vi "Remote Access.vi"() -> ()   [LabVIEW 2020, in "Startup Processes.lvlib"]
uses:
  Startup Processes.lvlib
  toolbox/Standard Signalling/ude_Stop Application/ude_Stop Application.lvlib
  toolbox/Standard Signalling/ude_Handle Errors/ude_Handle Errors.lvlib
  _ude/Read Graph Data/Read Graph Data.lvlib
  toolbox/Standard Signalling/not_Generic Named Notifier/not_Generic Named Notifier.lvlib
  _buffers/Sine Signal Data Buffer/Sine Signal Data Buffer.lvlib
  _buffers/Ramp Signal Data Buffer/Ramp Signal Data Buffer.lvlib
  _buffers/Temperature Controller Data Buffer/Temperature Controller Data Buffer.lvlib
  _ude/Read Graph Image/Read Graph Image.lvlib
  _buffers/Plugin Chart References/Plugin Chart References.lvlib
  _ude/Set Acquisition Rate/Set Acquisition Rate.lvlib
  _buffers/Sample Rate/Sample Rate.lvlib
  _ude/Set Data Buffer Depth/Set Data Buffer Depth.lvlib
  _ude/Set TC Parameters/Set TC Parameters.lvlib
  Config Data/Config Data.lvclass
  _typedefs/Pass Fail Flag.ctl
  _typedefs/Subpanel Names.ctl
panel:
  out "Last Event":string
  out "Last Plugin Name":T1
  out "Last Notifier":string
  out "Error Out":errorcluster
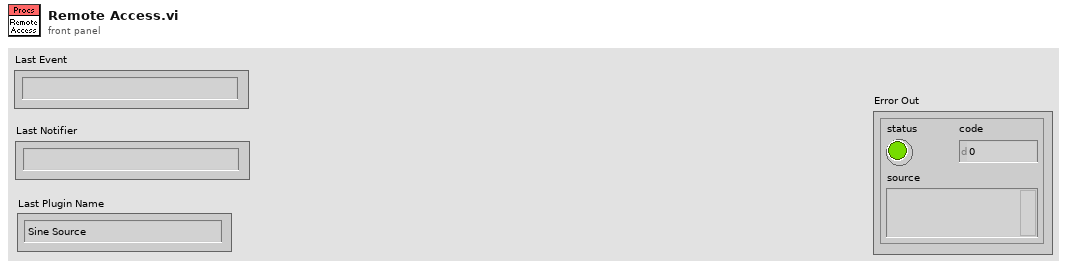
[diagram p1: front panel]
types:
  T1 = typedef "Startup Processes.lvlib/Subpanel Names.ctl" = enum16{"Sine Source", "Ramp Source", "Hen House TC", "Dog House TC", "Out House TC"}
  T2 = cluster{"sys":refnum<event-registration>, "RmtAcc":refnum<event-registration>, "RmtAcc":refnum<event-registration>, "RmtAcc":refnum<event-registration>, "RmtAcc":refnum<event-registration>, "RmtAcc":refnum<event-registration>}
  T3 = typedef "Startup Processes.lvlib/Pass Fail Flag.ctl" = enum16{"Update Good", "Update Failed"}
  T4 = typedef "Startup Processes.lvlib/Name Valid Flag.ctl" = enum16{"Name Valid", "Name Not Valid"}
  T5 = cluster{"Last value":dbl, "Error High Level":dbl, "Warning High Level":dbl, "Warning Low Level":dbl, "Error Low Level":dbl}[]
  T6 = typedef "imagedata.ctl" = cluster{"image type":i32, "image depth":i32, "image":u8[], "mask":u8[], "colors":u32[], "Rectangle":cluster{"left":i16, "top":i16, "right":i16, "bottom":i16}}
  T7 = typedef "Startup Processes.lvlib/TC Setup Parameters.ctl" = cluster{"Error High Level":dbl, "Warning High Level":dbl, "Warning Low Level":dbl, "Error Low Level":dbl, "Sample Interval":dbl[unit]}
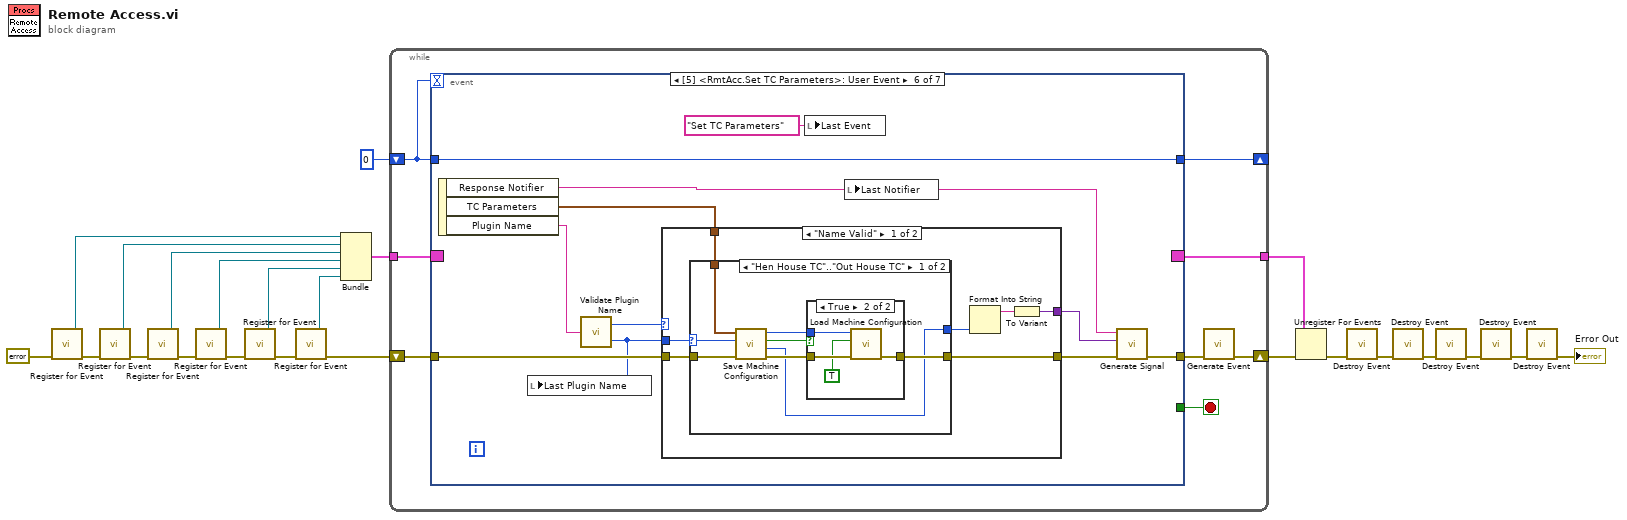
[diagram p0: block diagram]
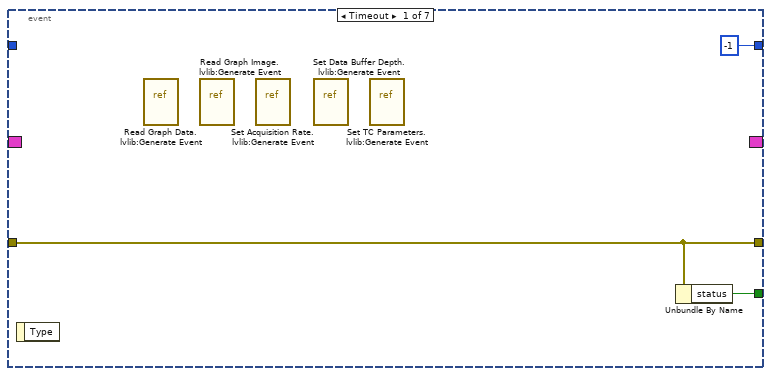
[diagram p2: hidden frame]
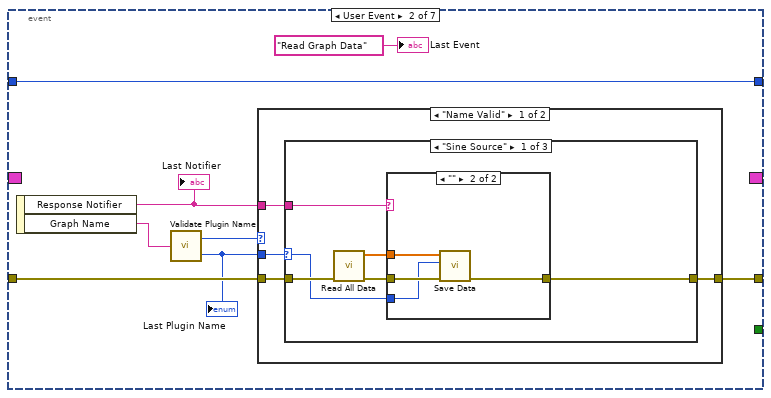
[diagram p3: hidden frame]
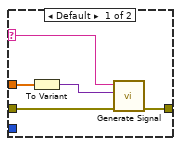
[diagram p4: hidden frame]
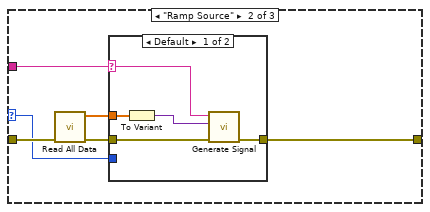
[diagram p5: hidden frame]
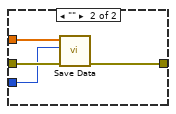
[diagram p6: hidden frame]
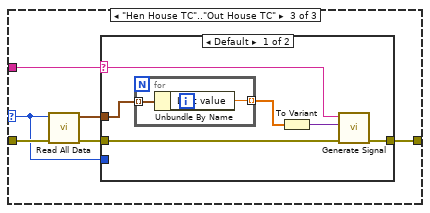
[diagram p7: hidden frame]
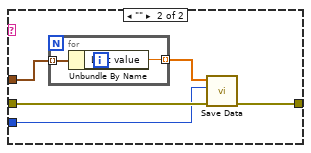
[diagram p8: hidden frame]
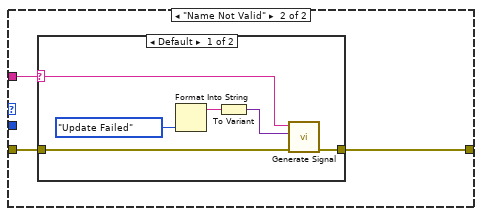
[diagram p9: hidden frame]
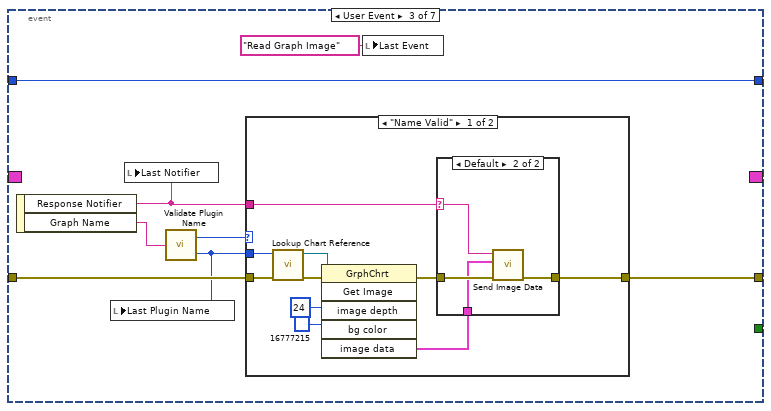
[diagram p11: hidden frame]
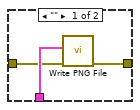
[diagram p12: hidden frame]
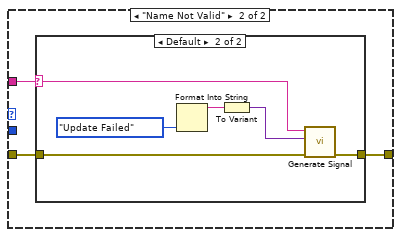
[diagram p13: hidden frame]
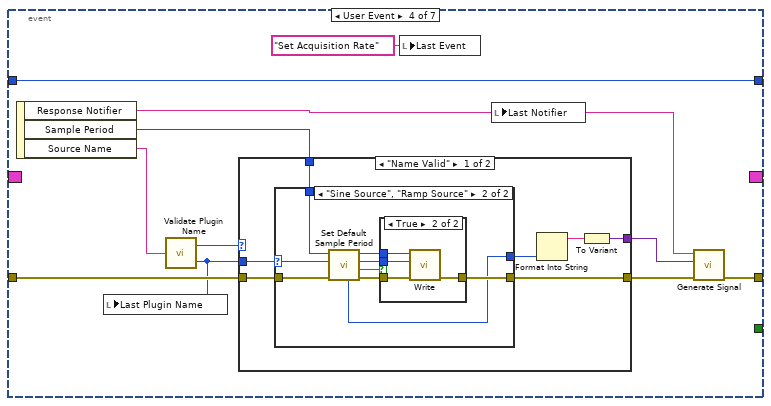
[diagram p15: hidden frame]
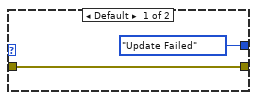
[diagram p16: hidden frame]
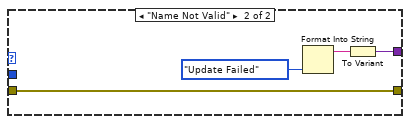
[diagram p18: hidden frame]
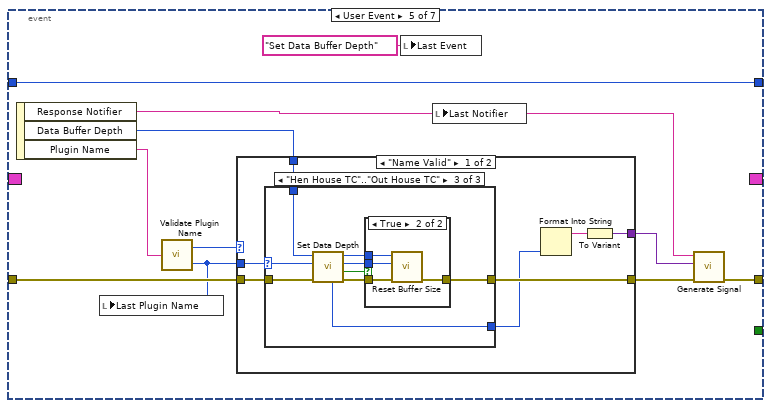
[diagram p19: hidden frame]
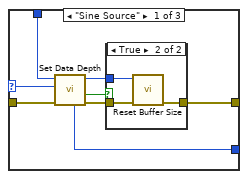
[diagram p20: hidden frame]
diagram:
  n1 = call "Register for Event.vi"("Error In"=errorcluster {"status"=FALSE, "code"=0, "source"=""} ("Error Out")) -> ("Error Out"=w18:errorcluster, "sys"=w22:refnum<event-registration>)  [unwired: 5 in]
  n2 = call "Register for Event.vi"("Error In"=w18) -> ("Error Out"=w17:errorcluster, "RmtAcc"=w19:refnum<event-registration>)  [unwired: 5 in]
  n3 = call "Register for Event.vi"("Error In"=w17) -> ("Error Out"=w11:errorcluster, "RmtAcc"=w16:refnum<event-registration>)  [unwired: 5 in]
  n4 = call "Register for Event.vi"("Error In"=w11) -> ("Error Out"=w7:errorcluster, "RmtAcc"=w12:refnum<event-registration>)  [unwired: 5 in]
  n5 = call "Register for Event.vi"("Error In"=w7) -> ("Error Out"=w4:errorcluster, "RmtAcc"=w8:refnum<event-registration>)  [unwired: 5 in]
  n6 = call "Register for Event.vi"("Error In"=w4) -> ("Error Out"=w3:errorcluster, "RmtAcc"=w2:refnum<event-registration>)  [unwired: 5 in]
  n7 = Bundle("sys"=w22, "RmtAcc"=w19, "RmtAcc"=w16, "RmtAcc"=w12, "RmtAcc"=w8, "RmtAcc"=w2) -> (w20:T2)  [unwired: 1 in]
  n8 = while {
    shift-right: [w27] -> w23
    shift-left: w3 -> [w31]
    tunnel: w20 -> [w30]
    tunnel: [w29] -> w15
    shift-right: [w24] -> _
    shift-left: 0 ("milliseconds to wait") -> [w25]
    stop <- w28 stop-if-true
    # "``"
    n9 = event shown="[5] <RmtAcc.Set TC Parameters>: User Event" {
      selector: w30 -> [_ _ _ _ _ _ _]
      dyn-events: [_ _ _ _ _ _ _] -> w29
      timeout: w25 -> [_ _ _ _ _ _ _]
      tunnel: w31 -> [w34 w41 w114 w150 w188 w248 w280]
      tunnel: [w34 w40 w111 w152 w190 w250 w280] -> w26
      tunnel: [w32 _ _ _ _ _ TRUE] -> w28
      tunnel: w25 -> [_ w42 w115 w153 w191 w251 w278]
      tunnel: [-1 ("milliseconds to wait") w42 w115 w153 w191 w251 w278] -> w24
      event Timeout {
        n10 = event-data() -> ()  [unwired: 1 in, 1 out]
        n11 = vi-ref "Read Graph Data.lvlib:Generate Event.vi"() -> ()  [unwired: 1 out]
        n12 = vi-ref "Read Graph Image.lvlib:Generate Event.vi"() -> ()  [unwired: 1 out]
        n13 = vi-ref "Set Acquisition Rate.lvlib:Generate Event.vi"() -> ()  [unwired: 1 out]
        n14 = vi-ref "Set Data Buffer Depth.lvlib:Generate Event.vi"() -> ()  [unwired: 1 out]
        n15 = vi-ref "Set TC Parameters.lvlib:Generate Event.vi"() -> ()  [unwired: 1 out]
        n16 = Unbundle By Name(w34) -> ("status"=w32:bool)
      }
      event User Event {
        n17 = event-data() -> ("Response Notifier"=w35:string, "Graph Name"=w39:string)  [unwired: 1 in]
        "Last Notifier" <- w35
        n18 = call "Validate Plugin Name.vi"("Name Input"=w39) -> ("Comparison Result"=w38:T4, "Plugin Name"=w36:T1)
        "Last Plugin Name" <- w36
        n19 = case shown="\"Name Valid\"" w38 {
          tunnel: w41 -> [w46 w100]
          tunnel: [w45 w99] -> w40
          tunnel: w35 -> [w44 w98]
          tunnel: w36 -> [w43 _]
          frame "Name Valid" {
            n20 = case shown="\"Sine Source\"" w43 {
              selector: w43 -> [w48 w63 w77]
              tunnel: w46 -> [w52 w67 w82]
              tunnel: [w49 w65 w80] -> w45
              tunnel: w44 -> [w47 w64 w79]
              frame "Sine Source" {
                n21 = call "Read All Data.vi"("Error In"=w52) -> ("Error Out"=w50:errorcluster, "Sine Data"=w51:dbl[])  [unwired: 5 in]
                n22 = case shown="\"\"" w47 {
                  selector: w47 -> [w56 _]
                  tunnel: w51 -> [w53 w61]
                  tunnel: w50 -> [w57 w60]
                  tunnel: [w55 w59] -> w49
                  tunnel: w48 -> [_ w58]
                  frame Default {
                    n23 = To Variant(anything=w53) -> (Variant=w54:variant)
                    n24 = call "Generate Signal.vi"("Error In"=w57, "Signal Data"=w54, "Notifier Name"=w56) -> ("Error Out"=w55:errorcluster)  [unwired: 4 in]
                  }
                  frame "" {
                    n25 = call "Save Data.vi"("error in (no error)"=w60, "My Name"=w58, "History Data"=w61) -> ("error out"=w59:errorcluster)  [unwired: 4 in]
                  }
                }
              }
              frame "Ramp Source" {
                n26 = call "Read All Data.vi"("Error In"=w67) -> ("Error Out"=w66:errorcluster, "Ramp Data"=w62:dbl[])  [unwired: 5 in]
                n27 = case shown="Default" w64 {
                  selector: w64 -> [w71 _]
                  tunnel: w62 -> [w68 w76]
                  tunnel: w66 -> [w72 w75]
                  tunnel: [w70 w74] -> w65
                  tunnel: w63 -> [_ w73]
                  frame Default {
                    n28 = To Variant(anything=w68) -> (Variant=w69:variant)
                    n29 = call "Generate Signal.vi"("Error In"=w72, "Signal Data"=w69, "Notifier Name"=w71) -> ("Error Out"=w70:errorcluster)  [unwired: 4 in]
                  }
                  frame "" {
                    n30 = call "Save Data.vi"("error in (no error)"=w75, "My Name"=w73, "History Data"=w76) -> ("error out"=w74:errorcluster)  [unwired: 4 in]
                  }
                }
              }
              frame "Hen House TC".."Out House TC" {
                n31 = call "Read All Data.vi"("Error In"=w82, "Instance Name"=w77) -> ("Error Out"=w81:errorcluster, "TC Data"=w78:T5)  [unwired: 4 in]
                n32 = case shown="Default" w79 {
                  selector: w79 -> [w87 _]
                  tunnel: w78 -> [w84 w91]
                  tunnel: w81 -> [w88 w95]
                  tunnel: [w86 w94] -> w80
                  tunnel: w77 -> [_ w93]
                  frame Default {
                    n33 = for {
                      tunnel: [w90] -> w83 mode=indexing
                      tunnel: w84 -> [w89] mode=indexing
                      n34 = Unbundle By Name(w89) -> ("Last value"=w90:dbl)
                    }
                    n35 = To Variant(anything=w83) -> (Variant=w85:variant)
                    n36 = call "Generate Signal.vi"("Error In"=w88, "Signal Data"=w85, "Notifier Name"=w87) -> ("Error Out"=w86:errorcluster)  [unwired: 4 in]
                  }
                  frame "" {
                    n37 = for {
                      tunnel: [w97] -> w92 mode=indexing
                      tunnel: w91 -> [w96] mode=indexing
                      n38 = Unbundle By Name(w96) -> ("Last value"=w97:dbl)
                    }
                    n39 = call "Save Data.vi"("error in (no error)"=w95, "My Name"=w93, "History Data"=w92) -> ("error out"=w94:errorcluster)  [unwired: 4 in]
                  }
                }
              }
            }
          }
          frame "Name Not Valid" {
            n40 = case shown="Default" w98 {
              selector: w98 -> [w105 _]
              tunnel: w100 -> [w106 w107]
              tunnel: [w104 w107] -> w99
              frame Default {
                n41 = Format Into String(Pass_Fail_Flag."Update Failed" ("Result")) -> (resulting string=w101:string)  [unwired: 3 in, 1 out]
                n42 = To Variant(anything=w101) -> (Variant=w103:variant)
                n43 = call "Generate Signal.vi"("Error In"=w106, "Signal Data"=w103, "Notifier Name"=w105) -> ("Error Out"=w104:errorcluster)  [unwired: 4 in]
              }
              frame "" {
              }
            }
          }
        }
        "Last Event" <- "Read Graph Data" ("Last Event")
      }
      event User Event {
        n44 = event-data() -> ("Response Notifier"=w110:string, "Graph Name"=w112:string)  [unwired: 1 in]
        n45 = local write "Last Notifier"(w110) -> ()
        n46 = call "Validate Plugin Name.vi"("Name Input"=w112) -> ("Comparison Result"=w113:T4, "Plugin Name"=w109:T1)
        n47 = local write "Last Plugin Name"(w109) -> ()
        n48 = case shown="\"Name Valid\"" w113 {
          tunnel: w114 -> [w124 w134]
          tunnel: [w117 w133] -> w111
          tunnel: w109 -> [w125 _]
          tunnel: w110 -> [w116 w135]
          frame "Name Valid" {
            n49 = call "Lookup Chart Reference.vi"("Error In"=w124, "Plugin Name"=w125) -> ("Error Out"=w123:errorcluster, "Reference Out"=w122:refnum<vi>)  [unwired: 4 in]
            n50 = invoke class="GrphChrt" method="Get Image"(reference=w122, error in=w123, "image depth"=24 ("Image Depth"), "bg color"=u32 16777215) -> (error out=w119:errorcluster, "image data"=w118:T6)  [unwired: 2 in, 4 out]
            n51 = case shown="Default" w116 {
              selector: w116 -> [_ w129]
              tunnel: w119 -> [w127 w132]
              tunnel: w118 -> [w128 w131]
              tunnel: [w126 w130] -> w117
              frame "" {
                n52 = call <vilib>:"Write PNG File.vi"("error in (no error)"=w127, "image data"=w128) -> ("error out"=w126:errorcluster)  [unwired: 8 in, 1 out]
              }
              frame Default {
                n53 = call "Send Image Data.vi"("error in (no error)"=w132, "image data"=w131, "Response Notifier"=w129) -> ("error out"=w130:errorcluster)  [unwired: 4 in]
              }
            }
          }
          frame "Name Not Valid" {
            n54 = case shown="Default" w135 {
              selector: w135 -> [_ w141]
              tunnel: w134 -> [w136 w140]
              tunnel: [w136 w139] -> w133
              frame "" {
              }
              frame Default {
                n55 = Format Into String(Pass_Fail_Flag."Update Failed" ("Result")) -> (resulting string=w137:string)  [unwired: 3 in, 1 out]
                n56 = To Variant(anything=w137) -> (Variant=w142:variant)
                n57 = call "Generate Signal.vi"("Error In"=w140, "Signal Data"=w142, "Notifier Name"=w141) -> ("Error Out"=w139:errorcluster)  [unwired: 4 in]
              }
            }
          }
        }
        n58 = local write "Last Event"("Read Graph Image" ("Last Event")) -> ()
      }
      event User Event {
        n59 = event-data() -> ("Response Notifier"=w145:string, "Sample Period"=w148:i32, "Source Name"=w146:string)  [unwired: 1 in]
        n60 = call "Validate Plugin Name.vi"("Name Input"=w146) -> ("Comparison Result"=w147:T4, "Plugin Name"=w144:T1)
        n61 = local write "Last Plugin Name"(w144) -> ()
        n62 = case shown="\"Name Valid\"" w147 {
          tunnel: [w160 w179] -> w151
          tunnel: w150 -> [w158 w180]
          tunnel: [w157 w180] -> w149
          tunnel: w144 -> [w159 _]
          tunnel: w148 -> [w156 _]
          frame "Name Valid" {
            n63 = case shown="\"Sine Source\", \"Ramp Source\"" w159 {
              selector: w159 -> [_ w170]
              tunnel: w158 -> [w162 w169]
              tunnel: [w162 w164] -> w157
              tunnel: [Pass_Fail_Flag."Update Failed" ("Result") w163] -> w154
              tunnel: w156 -> [_ w171]
              frame Default {
              }
              frame "Sine Source", "Ramp Source" {
                n64 = call "Set Default Sample Period.vi"("Sample Period (msec)"=w171, "Plugin Name"=w170, "error in (no error)"=w169) -> ("Result"=w163:T3, "Sample Period (msec) out"=w167:i32, "Plugin Name out"=w166:T1, "Changed?"=w165:bool, "error out"=w168:errorcluster)  [unwired: 1 in]
                n65 = case shown="True" w165 {
                  tunnel: w168 -> [w172 w176]
                  tunnel: w167 -> [_ w174]
                  tunnel: w166 -> [_ w173]
                  tunnel: [w172 w175] -> w164
                  frame False {
                  }
                  frame True {
                    n66 = call "Write.vi"("Error In"=w176, "Plugin Name"=w173, "Sample Period (msec)"=w174) -> ("Error Out"=w175:errorcluster)  [unwired: 2 in, 2 out]
                  }
                }
              }
            }
            n67 = Format Into String(w154) -> (resulting string=w155:string)  [unwired: 3 in, 1 out]
            n68 = To Variant(anything=w155) -> (Variant=w160:variant)
          }
          frame "Name Not Valid" {
            n69 = Format Into String(Pass_Fail_Flag."Update Failed" ("Result")) -> (resulting string=w177:string)  [unwired: 3 in, 1 out]
            n70 = To Variant(anything=w177) -> (Variant=w179:variant)
          }
        }
        n71 = local write "Last Event"("Set Acquisition Rate" ("Last Event")) -> ()
        n72 = local write "Last Notifier"(w145) -> ()
        n73 = call "Generate Signal.vi"("Error In"=w149, "Signal Data"=w151, "Notifier Name"=w145) -> ("Error Out"=w152:errorcluster)  [unwired: 4 in]
      }
      event User Event {
        n74 = event-data() -> ("Response Notifier"=w183:string, "Data Buffer Depth"=w186:i32, "Plugin Name"=w184:string)  [unwired: 1 in]
        n75 = call "Validate Plugin Name.vi"("Name Input"=w184) -> ("Comparison Result"=w185:T4, "Plugin Name"=w182:T1)
        n76 = local write "Last Plugin Name"(w182) -> ()
        n77 = case shown="\"Name Valid\"" w185 {
          tunnel: [w198 w239] -> w189
          tunnel: w188 -> [w196 w240]
          tunnel: [w194 w240] -> w187
          tunnel: w182 -> [w197 _]
          tunnel: w186 -> [w195 _]
          frame "Name Valid" {
            n78 = case shown="\"Hen House TC\"..\"Out House TC\"" w197 {
              selector: w197 -> [w203 w216 w229]
              tunnel: w196 -> [w202 w215 w228]
              tunnel: [w206 w218 w231] -> w194
              tunnel: w195 -> [w205 w217 w230]
              tunnel: [w204 w212 w223] -> w192
              frame "Sine Source" {
                n79 = call "Set Data Depth.vi"("New Buffer Size"=w205, "Plugin Names"=w203, "error in (no error)"=w202) -> ("Result"=w204:T3, "New Buffer Size out"=w199:i32, "Changed?"=w200:bool, "error out"=w201:errorcluster)  [unwired: 1 in, 1 out]
                n80 = case shown="True" w200 {
                  tunnel: [w207 w208] -> w206
                  tunnel: w201 -> [w207 w209]
                  tunnel: w199 -> [_ w210]
                  frame False {
                  }
                  frame True {
                    n81 = call "Reset Buffer Size.vi"("Error In"=w209, "New Buffer Size"=w210) -> ("Error Out"=w208:errorcluster)  [unwired: 5 in]
                  }
                }
              }
              frame "Ramp Source" {
                n82 = call "Set Data Depth.vi"("New Buffer Size"=w217, "Plugin Names"=w216, "error in (no error)"=w215) -> ("Result"=w212:T3, "New Buffer Size out"=w213:i32, "Changed?"=w211:bool, "error out"=w214:errorcluster)  [unwired: 1 in, 1 out]
                n83 = case shown="True" w211 {
                  tunnel: w213 -> [_ w222]
                  tunnel: w214 -> [w219 w221]
                  tunnel: [w219 w220] -> w218
                  frame False {
                  }
                  frame True {
                    n84 = call "Reset Buffer Size.vi"("Error In"=w221, "New Buffer Size"=w222) -> ("Error Out"=w220:errorcluster)  [unwired: 5 in]
                  }
                }
              }
              frame "Hen House TC".."Out House TC" {
                n85 = call "Set Data Depth.vi"("New Buffer Size"=w230, "Plugin Names"=w229, "error in (no error)"=w228) -> ("Result"=w223:T3, "New Buffer Size out"=w227:i32, "Plugin Names out"=w226:T1, "Changed?"=w225:bool, "error out"=w224:errorcluster)  [unwired: 1 in]
                n86 = case shown="True" w225 {
                  tunnel: w224 -> [w232 w234]
                  tunnel: [w232 w233] -> w231
                  tunnel: w227 -> [_ w236]
                  tunnel: w226 -> [_ w235]
                  frame False {
                  }
                  frame True {
                    n87 = call "Reset Buffer Size.vi"("Error In"=w234, "Instance Name"=w235, "New Buffer Size"=w236) -> ("Error Out"=w233:errorcluster)  [unwired: 4 in]
                  }
                }
              }
            }
            n88 = Format Into String(w192) -> (resulting string=w193:string)  [unwired: 3 in, 1 out]
            n89 = To Variant(anything=w193) -> (Variant=w198:variant)
          }
          frame "Name Not Valid" {
            n90 = Format Into String(Pass_Fail_Flag."Update Failed" ("Result")) -> (resulting string=w237:string)  [unwired: 3 in, 1 out]
            n91 = To Variant(anything=w237) -> (Variant=w239:variant)
          }
        }
        n92 = local write "Last Event"("Set Data Buffer Depth" ("Last Event")) -> ()
        n93 = local write "Last Notifier"(w183) -> ()
        n94 = call "Generate Signal.vi"("Error In"=w187, "Signal Data"=w189, "Notifier Name"=w183) -> ("Error Out"=w190:errorcluster)  [unwired: 4 in]
      }
      event User Event {
        n95 = event-data() -> ("Response Notifier"=w243:string, "TC Parameters"=w246:T7, "Plugin Name"=w244:string)  [unwired: 1 in]
        n96 = call "Validate Plugin Name.vi"("Name Input"=w244) -> ("Comparison Result"=w245:T4, "Plugin Name"=w242:T1)
        n97 = local write "Last Plugin Name"(w242) -> ()
        n98 = case shown="\"Name Valid\"" w245 {
          tunnel: [w258 w276] -> w249
          tunnel: w248 -> [w256 w277]
          tunnel: [w254 w277] -> w247
          tunnel: w242 -> [w257 _]
          tunnel: w246 -> [w255 _]
          frame "Name Valid" {
            n99 = case shown="\"Hen House TC\"..\"Out House TC\"" w257 {
              selector: w257 -> [w265 _]
              tunnel: w256 -> [w264 w273]
              tunnel: [w261 w273] -> w254
              tunnel: w255 -> [w266 _]
              tunnel: [w259 Pass_Fail_Flag."Update Failed" ("Result")] -> w252
              frame "Hen House TC".."Out House TC" {
                n100 = call "Save Machine Configuration.vi"("error in (no error)"=w264, "Plugin Name"=w265, "TC Parameters"=w266) -> ("error out"=w263:errorcluster, "Result"=w259:T3, "Changed?"=w260:bool, "Plugin Name out"=w262:T1)  [unwired: 1 in]
                n101 = case shown="True" w260 {
                  tunnel: w263 -> [w267 w271]
                  tunnel: w262 -> [_ w270]
                  tunnel: [w267 w269] -> w261
                  frame False {
                  }
                  frame True {
                    n102 = call "Load Machine Configuration.vi"("error in (no error)"=w271, "Reload?"=TRUE, "Instance Name"=w270) -> ("error out"=w269:errorcluster)  [unwired: 3 in, 1 out]
                  }
                }
              }
              frame Default {
              }
            }
            n103 = Format Into String(w252) -> (resulting string=w253:string)  [unwired: 3 in, 1 out]
            n104 = To Variant(anything=w253) -> (Variant=w258:variant)
          }
          frame "Name Not Valid" {
            n105 = Format Into String(Pass_Fail_Flag."Update Failed" ("Result")) -> (resulting string=w274:string)  [unwired: 3 in, 1 out]
            n106 = To Variant(anything=w274) -> (Variant=w276:variant)
          }
        }
        n107 = local write "Last Event"("Set TC Parameters" ("Last Event")) -> ()
        n108 = local write "Last Notifier"(w243) -> ()
        n109 = call "Generate Signal.vi"("Error In"=w247, "Signal Data"=w249, "Notifier Name"=w243) -> ("Error Out"=w250:errorcluster)  [unwired: 4 in]
      }
      event User Event {
        n110 = event-data() -> ()  [unwired: 1 in, 1 out]
      }
    }
    n111 = call "Generate Event.vi"("Error In"=w26) -> ("Error Out"=w27:errorcluster)  [unwired: 6 in]
  }
  n112 = Unregister For Events(event registration refnum=w15, error in=w23) -> (error out=w14:errorcluster)
  n113 = call "Destroy Event.vi"("Error In"=w14) -> ("Error Out"=w13:errorcluster)  [unwired: 6 in]
  n114 = call "Destroy Event.vi"("Error In"=w13) -> ("Error Out"=w10:errorcluster)  [unwired: 6 in]
  n115 = call "Destroy Event.vi"("Error In"=w10) -> ("Error Out"=w9:errorcluster)  [unwired: 6 in]
  n116 = call "Destroy Event.vi"("Error In"=w9) -> ("Error Out"=w6:errorcluster)  [unwired: 6 in]
  n117 = call "Destroy Event.vi"("Error In"=w6) -> ("Error Out"=→"Error Out":errorcluster)  [unwired: 6 in]
